vi "Pneumatic gripper grab.vi"(8 "error in":errorcluster, 10 "pump  sec":dbl=0.8 format="%#_13g") -> (0 "error out":errorcluster)   [LabVIEW 2019]
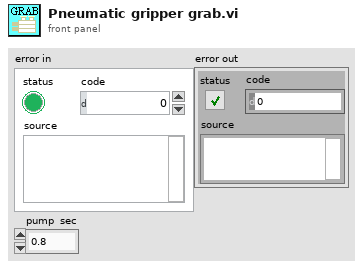
[diagram p1: front panel]
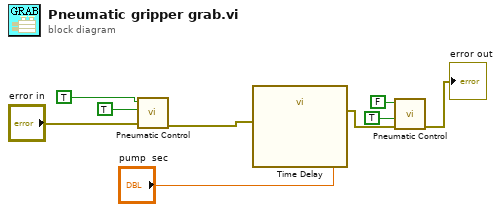
[diagram p0: block diagram]
diagram:
  n1 = call "Pneumatic Control.vi"("error in"="error in", "DIR"=TRUE, "ENA"=TRUE) -> ("error out"=w7:errorcluster)  [unwired: 8 in]
  n2 = call "Time Delay"("error in (no error)"=w7, "Delay Time (s)"="pump  sec") -> ("error out"=w5:errorcluster)  [unwired: 9 in]
  n3 = call "Pneumatic Control.vi"("error in"=w5, "DIR"=TRUE, "ENA"=FALSE) -> ("error out"=→"error out":errorcluster)  [unwired: 8 in]
